vi "DflipFlop_Fast.vi"(8 "D":bool, 9 "Clock":bool, 10 "Reset":bool, 11 "Set":bool) -> (2 "/Q\\":bool, 3 "Q":bool)   [LabVIEW 2012]
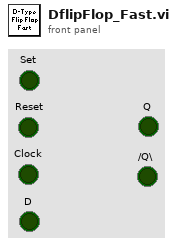
[diagram p1: front panel]
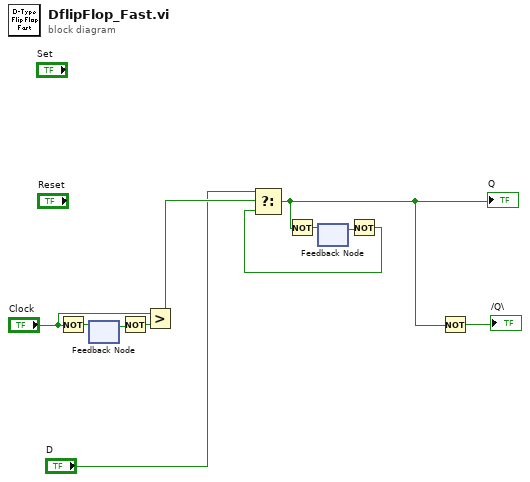
[diagram p0: block diagram]
diagram:
  n1 = Not(x="Clock") -> (.not. x?=w8:bool)
  n2 = feedback-in #1(w8) -> ()
  n3 = feedback #1() -> (w6:bool)  [unwired: 1 in]
  n4 = Not(x=w6) -> (.not. x?=w5:bool)
  n5 = Greater?(x="Clock", y=w5) -> (0:w11:bool)
  n6 = feedback #2() -> (w4:bool)  [unwired: 1 in]
  n7 = Not(x=w4) -> (.not. x?=w1:bool)
  n8 = Select(t="D", s=w11, f=w1) -> (s? t:f=w2:bool)
  "Q" <- w2
  n9 = Not(x=w2) -> (.not. x?=w3:bool)
  n10 = feedback-in #2(w3) -> ()
  n11 = Not(x=w2) -> (.not. x?=→"/Q\\":bool)
